vi "thrhand.vi"() -> (0 "b":cluster{"bmin":dbl, "bmax":dbl}, 1 "a":cluster{"amin":dbl, "amax":dbl}, 2 "L":cluster{"Lmin":dbl, "Lmax":dbl})   [LabVIEW 2018]
panel:
  in  "停止":bool
  in  "bmax":dbl
  in  "bmin":dbl
  in  "amax":dbl
  in  "amin":dbl
  in  "Lmax":dbl
  in  "Lmin":dbl
  # "请手动输入Lab的阈值"
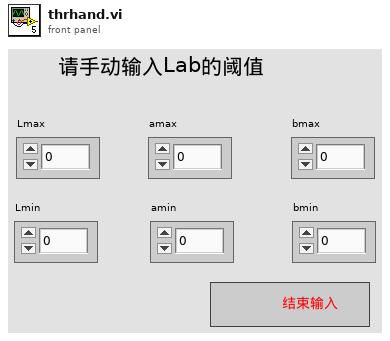
[diagram p1: front panel]
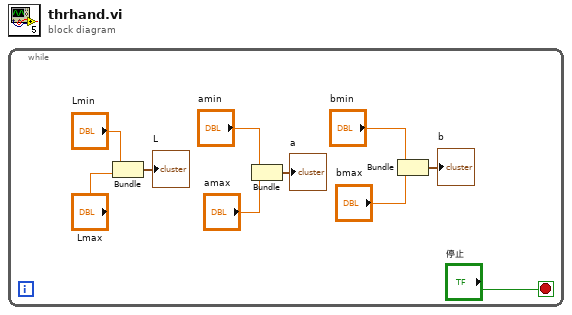
[diagram p0: block diagram]
diagram:
  n1 = while {
    stop <- "停止" stop-if-true
    n2 = Bundle("Lmin"="Lmin", "Lmax"="Lmax") -> (→"L":cluster{"Lmin":dbl, "Lmax":dbl})  [unwired: 1 in]
    n3 = Bundle("amin"="amin", "amax"="amax") -> (→"a":cluster{"amin":dbl, "amax":dbl})  [unwired: 1 in]
    n4 = Bundle("bmin"="bmin", "bmax"="bmax") -> (→"b":cluster{"bmin":dbl, "bmax":dbl})  [unwired: 1 in]
  }
